vi "fbd_test.vi"(1 "in":dbl) -> (0 "out":dbl)   [LabVIEW 2021]
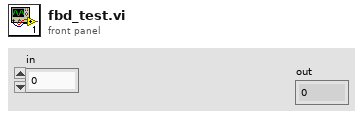
[diagram p1: front panel]
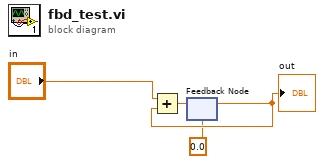
[diagram p0: block diagram]
diagram:
  n1 = feedback #1(0.0) -> (w2:dbl)
  "out" <- w2
  n2 = Add(x="in", y=w2) -> (x+y=w3:dbl)
  n3 = feedback-in #1(w3) -> ()
